vi "CRYMake Unity cal Step and unity dat.vi"(8 "Write?":bool=TRUE, 11 "Hardware flattened":string) -> (3 "Calibration flattened":string)   [LabVIEW 2013]
uses:
  Typedef Control/CRYCalibration All Cluster.ctl
  Typedef Control/CRYCalibration 2DCluster.ctl
  Typedef Control/CRYCalibration Cluster.ctl
  Typedef Control/CRYData Cluster.ctl
  CRYMainGlobal.vi
panel:
  out "output cluster":T1 {"Calibration 2D"."Sens Curve"."Z data" items=["dB", "Lin"]; "Calibration 2D"."Sens Curve"."X data" items=["dB", "Lin"]; "Calibration 2D"."Sens Curve"."Y data" items=["dB", "Lin"]; "Calibration 2D"."Sens Curve"."Z dB ref" format="%.1f"; "Calibration 2D"."Sens Curve"."Z axis" items=["Log", "Lin"]; "Calibration 2D"."Sens Curve"."X dB ref" format="%.1f"; "Calibration 2D"."Sens Curve"."X axis" items=["Log", "Lin"]; "Calibration 2D"."Sens Curve"."Y axis" items=["Log", "Lin"]; "Calibration 2D"."Sens Curve"."Y dB ref" format="%.1f"; "Calibration 2D"."Sens Curve"."Curve"."z" format="%.2f"; "Calibration 2D"."Sens Curve"."Curve"."y" format="%.2f"; "Calibration 2D"."Sens Curve"."Curve"."x" format="%.2f"; "Calibration 2D"."EQ Curve"."Z data" items=["dB", "Lin"]; "Calibration 2D"."EQ Curve"."X data" items=["dB", "Lin"]; "Calibration 2D"."EQ Curve"."Y data" items=["dB", "Lin"]; "Calibration 2D"."EQ Curve"."Z dB ref" format="%.1f"; "Calibration 2D"."EQ Curve"."Z axis" items=["Log", "Lin"]; "Calibration 2D"."EQ Curve"."X dB ref" format="%.1f"; "Calibration 2D"."EQ Curve"."X axis" items=["Log", "Lin"]; "Calibration 2D"."EQ Curve"."Y axis" items=["Log", "Lin"]; "Calibration 2D"."EQ Curve"."Y dB ref" format="%.1f"; "Calibration 2D"."EQ Curve"."Curve"."z" format="%.2f"; "Calibration 2D"."EQ Curve"."Curve"."y" format="%.2f"; "Calibration 2D"."EQ Curve"."Curve"."x" format="%.2f"; "Calibration 2D"."Corr Curve"."Z data" items=["dB", "Lin"]; "Calibration 2D"."Corr Curve"."X data" items=["dB", "Lin"]; "Calibration 2D"."Corr Curve"."Y data" items=["dB", "Lin"]; "Calibration 2D"."Corr Curve"."Z dB ref" format="%.1f"; "Calibration 2D"."Corr Curve"."Z axis" items=["Log", "Lin"]; "Calibration 2D"."Corr Curve"."X dB ref" format="%.1f"; "Calibration 2D"."Corr Curve"."X axis" items=["Log", "Lin"]; "Calibration 2D"."Corr Curve"."Y axis" items=["Log", "Lin"]; "Calibration 2D"."Corr Curve"."Y dB ref" format="%.1f"; "Calibration 2D"."Corr Curve"."Curve"."z" format="%.2f"; "Calibration 2D"."Corr Curve"."Curve"."y" format="%.2f"; "Calibration 2D"."Corr Curve"."Curve"."x" format="%.2f"; "Calibration 2D"."Calibration"."EQ Step size" items=["R10", "R20", "R40", "R80", "User"]; "Calibration 2D"."Calibration"."Corr Step size" items=["R10", "R20", "R40", "R80", "User"]}
  out "OK?":bool
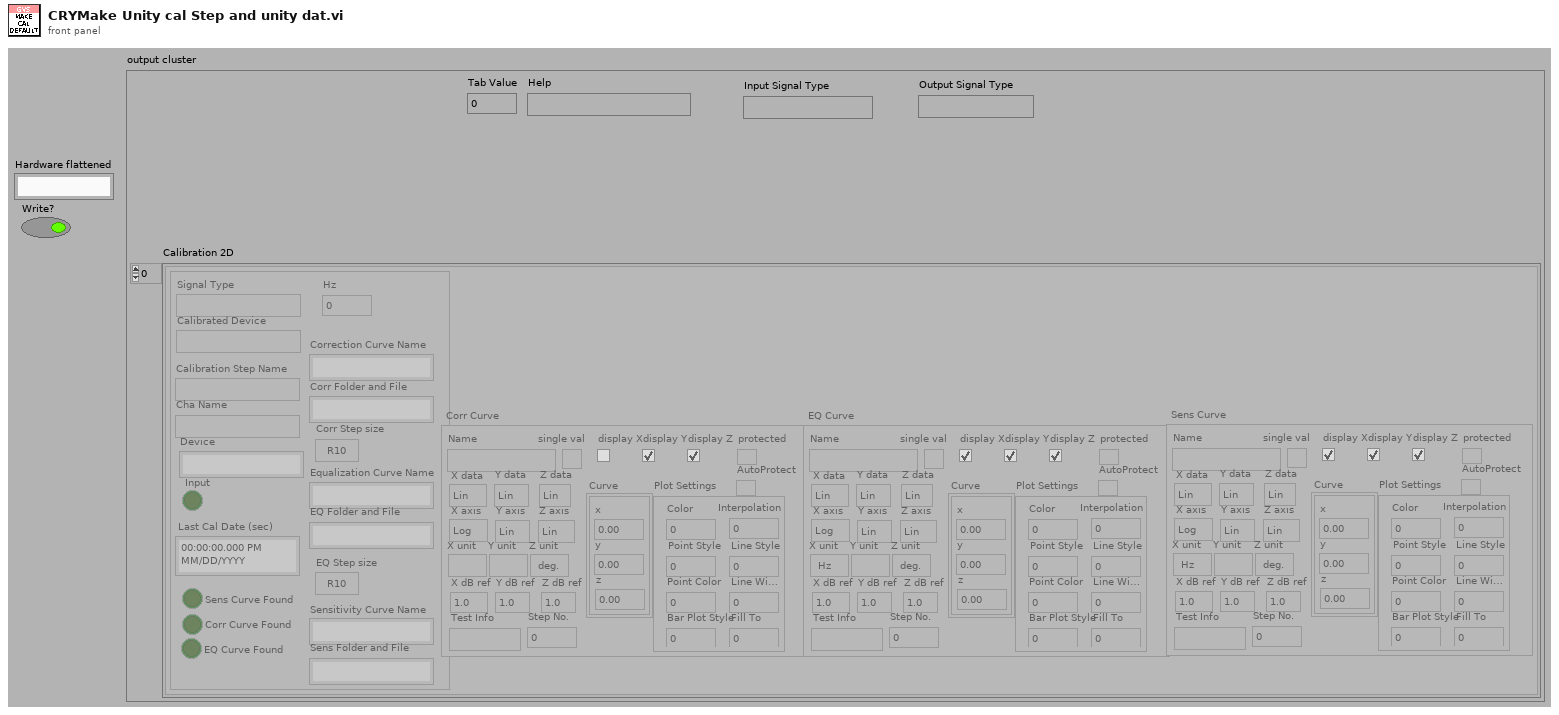
[diagram p1: front panel]
types:
  T1 = typedef "CRYCalibration All Cluster.ctl" = cluster{"Calibration 2D":T2[], "Help":string, "Tab Value":i32, "Input Signal Type":string, "Output Signal Type":string}
  T2 = typedef "CRYCalibration 2DCluster.ctl" = cluster{"Calibration":T3, "Corr Curve":T4, "EQ Curve":T4, "Sens Curve":T4}
  T3 = typedef "CRYCalibration Cluster.ctl" = cluster{"Calibration Step Name":string, "Device":string, "Correction Curve Name":string, "Equalization Curve Name":string, "Sensitivity Curve Name":string, "Corr Folder and File":string, "EQ Folder and File":string, "Sens Folder and File":string, "Corr Step size":u16, "EQ Step size":u16, "Input":bool, "Last Cal Date (sec)":timestamp, "Cha Name":string, "Corr Curve Found":bool, "EQ Curve Found":bool, "Sens Curve Found":bool, "Signal Type":string, "Calibrated Device":string, "Hz":u32}
  T4 = typedef "CRYData Cluster.ctl" = cluster{"Name":string, "Curve":cluster{"x":dbl, "y":dbl, "z":dbl}[], "X data":u16, "Y data":u16, "Z data":u16, "X axis":u16, "Y axis":u16, "Z axis":u16, "X unit":string, "Y unit":string, "Z unit":string, "X dB ref":dbl, "Y dB ref":dbl, "Z dB ref":dbl, "single val":bool, "protected":bool, "display X":bool, "display Y":bool, "display Z":bool, "Test Info":string, "Step No.":i32, "Plot Settings":cluster{"Color":u32, "Interpolation":u8, "Point Style":u8, "Line Style":u8, "Point Color":u32, "Line Width":u8, "Bar Plot Style":u8, "Fill To":i16}, "AutoProtect":bool}
  T5 = cluster{"StepName":string, "setup flattened":string}[]
  T6 = cluster{"StepName":string, "setup flattened":string}
  T7 = enum16{"open", "replace", "create", "open or create", "replace or create", "replace or create with confirmation"}
  T8 = enum16{"big-endian, network order", "native, host order", "little-endian"}
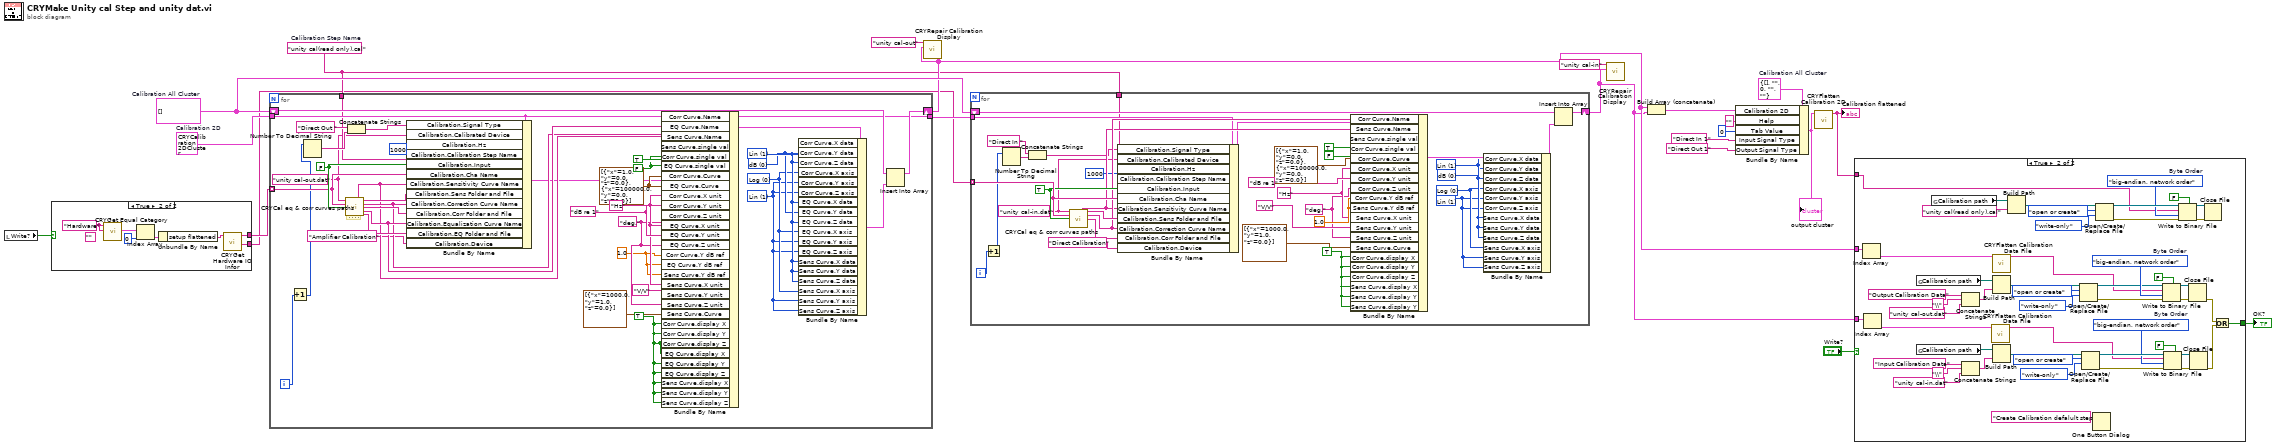
[diagram p0: block diagram]
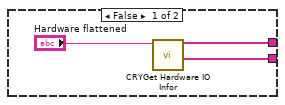
[diagram p2: hidden frame]
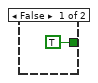
[diagram p3: hidden frame]
diagram:
  w5 = "unity cal(read only).cal"  # Calibration Step Name
  w19 = T1 {"Calibration 2D"=[], "Help"="", "Tab Value"=0, "Input Signal Type"="", "Output Signal Type"=""}  # Calibration All Cluster
  w20 = T2 {"Calibration"={"Calibration Step Name"="", "Device"="", "Correction Curve Name"="", "Equalization Curve Name"="", "Sensitivity Curve Name"="", "Corr Folder and File"="", "EQ Folder and File"="", "Sens Folder and File"="", "Corr Step size"=0, "EQ Step size"=0, "Input"=FALSE, "Last Cal Date (sec)"=timestamp(0 s since 1904-01-01), "Cha Name"="", "Corr Curve Found"=FALSE, "EQ Curve Found"=FALSE, "Sens Curve Found"=FALSE, "Signal Type"="", "Calibrated Device"="", "Hz"=0}, "Corr Curve"={"Name"="", "Curve"=[], "X data"=1, "Y data"=1, "Z data"=1, "X axis"=0, "Y axis"=1, "Z axis"=1, "X unit"="", "Y unit"="", "Z unit"="deg.", "X dB ref"=1.0, "Y dB ref"=1.0, "Z dB ref"=1.0, "single val"=FALSE, "protected"=FALSE, "display X"=FALSE, "display Y"=TRUE, "display Z"=TRUE, "Test Info"="", "Step No."=0, "Plot Settings"={"Color"=0, "Interpolation"=0, "Point Style"=0, "Line Style"=0, "Point Color"=0, "Line Width"=0, "Bar Plot Style"=0, "Fill To"=0}, "AutoProtect"=FALSE}, "EQ Curve"={"Name"="", "Curve"=[], "X data"=1, "Y data"=1, "Z data"=1, "X axis"=0, "Y axis"=1, "Z axis"=1, "X unit"="Hz", "Y unit"="", "Z unit"="deg.", "X dB ref"=1.0, "Y dB ref"=1.0, "Z dB ref"=1.0, "single val"=FALSE, "protected"=FALSE, "display X"=TRUE, "display Y"=TRUE, "display Z"=TRUE, "Test Info"="", "Step No."=0, "Plot Settings"={"Color"=0, "Interpolation"=0, "Point Style"=0, "Line Style"=0, "Point Color"=0, "Line Width"=0, "Bar Plot Style"=0, "Fill To"=0}, "AutoProtect"=FALSE}, "Sens Curve"={"Name"="", "Curve"=[], "X data"=1, "Y data"=1, "Z data"=1, "X axis"=0, "Y axis"=1, "Z axis"=1, "X unit"="Hz", "Y unit"="", "Z unit"="deg.", "X dB ref"=1.0, "Y dB ref"=1.0, "Z dB ref"=1.0, "single val"=FALSE, "protected"=FALSE, "display X"=TRUE, "display Y"=TRUE, "display Z"=TRUE, "Test Info"="", "Step No."=0, "Plot Settings"={"Color"=0, "Interpolation"=0, "Point Style"=0, "Line Style"=0, "Point Color"=0, "Line Width"=0, "Bar Plot Style"=0, "Fill To"=0}, "AutoProtect"=FALSE}}  # Calibration 2D
  w9 = T2[] []  # Calibration All Cluster
  n1 = local read "Write?"() -> (w3:bool)
  n2 = case shown="True" w3 {
    tunnel: [w23 w27] -> w2
    tunnel: [w22 w26] -> w1
    frame False {
      n3 = call "CRYGet Hardware IO Infor.vi"("Hardware setup In"="Hardware flattened") -> ("I_Hardware Channel Name Out"=w22:string[], "O_Hardware Channel Name Out"=w23:string[])  [unwired: 9 out]
    }
    frame True {
      (unwired) ""
      w25 = "Hardware" ("CategoryName")
      n4 = call "CRYGet Equal Category.vi"("Current StepName"=w25, "Find CategoryName"=w25) -> ("setup flattened Array out"=w29:T5)  [unwired: 9 out]
      n5 = Index Array(array=w29, index=0) -> (element=w30:T6)
      n6 = Unbundle By Name(w30) -> ("setup flattened"=w31:string)
      n7 = call "CRYGet Hardware IO Infor.vi"("Hardware setup In"=w31) -> ("I_Hardware Channel Name Out"=w26:string[], "O_Hardware Channel Name Out"=w27:string[])  [unwired: 9 out]
    }
  }
  n8 = for {
    tunnel: w2 -> [w37] mode=indexing
    shift-right: [w42] -> w7
    shift-left: w9 -> [w43]
    tunnel: w20 -> [w41]
    tunnel: [w41] -> w21
    tunnel: w5 -> [w33]
    i -> [w36]
    w32 = "unity cal-out.dat" ("Step Name")
    w48 = u16 1 items=["Log", "Lin"] ("Y axis")
    w49 = u16 0 items=["Log", "Lin"] ("Y axis")
    w50 = u16 0 items=["dB", "Lin"] ("Y data")
    w51 = u16 1 items=["dB", "Lin"] ("Y data")
    w52 = TRUE ("Corr Curve.display X")
    w58 = 1.0 ("EQ Curve.Y dB ref")
    w59 = "deg." ("Corr Curve.Z unit")
    w62 = "dB re 1" ("Corr Curve.Y unit")
    w61 = "Hz" ("Corr Curve.X unit")
    w63 = cluster{"x":dbl, "y":dbl, "z":dbl}[] [{"x"=1.0, "y"=0.0, "z"=0.0}, {"x"=100000.0, "y"=0.0, "z"=0.0}] ("Corr Curve.Curve")
    w64 = FALSE ("Corr Curve.single val")
    w68 = FALSE ("Input")
    # "????"
    n9 = Increment(x=w36) -> (x+1=w34:i32)
    n10 = Number To Decimal String(number=w34) -> (decimal integer string=w35:string)  [unwired: 1 in]
    n11 = call "CRYCal eq & corr curves paths.vi"("Calibrated Device Name"=w32, "Channel Name"=w37, "In_Out"=w68) -> ("Sens Currve Name"=w53:string, "Sens Curve File"=w67:string, "Corr Curve Name"=w54:string, "Corr Curve File"=w56:string, "EQ Curve Name"=w55:string, "EQ Curve File"=w66:string)  [unwired: 7 out]
    n12 = Concatenate Strings("Direct Out " ("Calibration.Signal Type"), w35) -> (w38:string)
    n13 = Bundle By Name(cluster=w41, "Calibration.Signal Type"=w38, "Calibration.Calibrated Device"=w32, "Calibration.Hz"=u32 1000, "Calibration.Calibration Step Name"=w33, "Calibration.Input"=w68, "Calibration.Cha Name"=w37, "Calibration.Sensitivity Curve Name"=w53, "Calibration.Sens Folder and File"=w67, "Calibration.Correction Curve Name"=w54, "Calibration.Corr Folder and File"=w56, "Calibration.Equalization Curve Name"=w55, "Calibration.EQ Folder and File"=w66, "Calibration.Device"="Amplifier Calibration" ("Device")) -> (w46:T2)
    n14 = Bundle By Name(cluster=w46, "Corr Curve.Name"=w54, "EQ Curve.Name"=w55, "Sens Curve.Name"=w53, "Sens Curve.single val"=TRUE, "Corr Curve.single val"=w64, "EQ Curve.single val"=w64, "Corr Curve.Curve"=w63, "EQ Curve.Curve"=w63, "Corr Curve.X unit"=w61, "Corr Curve.Y unit"=w62, "Corr Curve.Z unit"=w59, "EQ Curve.X unit"=w61, "EQ Curve.Y unit"=w62, "EQ Curve.Z unit"=w59, "Corr Curve.Y dB ref"=w58, "EQ Curve.Y dB ref"=w58, "Sens Curve.Y dB ref"=w58, "Sens Curve.X unit"=w61, "Sens Curve.Y unit"="V/V", "Sens Curve.Z unit"=w59, "Sens Curve.Curve"=cluster{"x":dbl, "y":dbl, "z":dbl}[] [{"x"=1000.0, "y"=1.0, "z"=0.0}], "Corr Curve.display X"=w52, "Corr Curve.display Y"=w52, "Corr Curve.display Z"=w52, "EQ Curve.display X"=w52, "EQ Curve.display Y"=w52, "EQ Curve.display Z"=w52, "Sens Curve.display X"=w52, "Sens Curve.display Y"=w52, "Sens Curve.display Z"=w52) -> (w45:T2)
    n15 = Bundle By Name(cluster=w45, "Corr Curve.X data"=w51, "Corr Curve.Y data"=w50, "Corr Curve.Z data"=w51, "Corr Curve.X axis"=w49, "Corr Curve.Y axis"=w48, "Corr Curve.Z axis"=w48, "EQ Curve.X data"=w51, "EQ Curve.Y data"=w50, "EQ Curve.Z data"=w51, "EQ Curve.X axis"=w49, "EQ Curve.Y axis"=w48, "EQ Curve.Z axis"=w48, "Sens Curve.X data"=w51, "Sens Curve.Y data"=w51, "Sens Curve.Z data"=w51, "Sens Curve.X axis"=w49, "Sens Curve.Y axis"=w48, "Sens Curve.Z axis"=w48) -> (w44:T2)
    n16 = Insert Into Array(array=w43, new element=w44) -> (w42:T2[])  [unwired: 1 in]
  }
  n17 = call "CRYRepair Calibration Display.vi"("Calibration In"=w7, "Calibration Step Name"="unity cal-out") -> ()  [unwired: 1 in, 9 out]
  n18 = for {
    tunnel: w1 -> [w103] mode=indexing
    tunnel: w21 -> [w81]
    shift-right: [w78] -> w6
    shift-left: w9 -> [w79]
    tunnel: w5 -> [w70]
    i -> [w76]
    w69 = "unity cal-in.dat" ("Step Name")
    w83 = u16 1 items=["Log", "Lin"] ("Y axis")
    w84 = u16 0 items=["Log", "Lin"] ("Y axis")
    w85 = u16 0 items=["dB", "Lin"] ("Y data")
    w86 = u16 1 items=["dB", "Lin"] ("Y data")
    w88 = TRUE ("Corr Curve.display X")
    w95 = 1.0 ("EQ Curve.Y dB ref")
    w92 = "deg." ("Corr Curve.Z unit")
    w94 = "Hz" ("Corr Curve.X unit")
    w102 = TRUE ("Input")
    n19 = Increment(x=w76) -> (x+1=w71:i32)
    n20 = Number To Decimal String(number=w71) -> (decimal integer string=w75:string)  [unwired: 1 in]
    n21 = Concatenate Strings("Direct In " ("string"), w75) -> (w72:string)
    n22 = call "CRYCal eq & corr curves paths.vi"("Calibrated Device Name"=w69, "Channel Name"=w103, "In_Out"=w102) -> ("Sens Currve Name"=w89:string, "Sens Curve File"=w101:string, "Corr Curve Name"=w90:string, "Corr Curve File"=w100:string)  [unwired: 9 out]
    n23 = Bundle By Name(cluster=w81, "Calibration.Signal Type"=w72, "Calibration.Calibrated Device"=w69, "Calibration.Hz"=u32 1000, "Calibration.Calibration Step Name"=w70, "Calibration.Input"=w102, "Calibration.Cha Name"=w103, "Calibration.Sensitivity Curve Name"=w89, "Calibration.Sens Folder and File"=w101, "Calibration.Correction Curve Name"=w90, "Calibration.Corr Folder and File"=w100, "Calibration.Device"="Direct Calibration" ("Device")) -> (w80:T2)
    n24 = Bundle By Name(cluster=w80, "Corr Curve.Name"=w90, "Sens Curve.Name"=w89, "Sens Curve.single val"=TRUE, "Corr Curve.single val"=FALSE, "Corr Curve.Curve"=cluster{"x":dbl, "y":dbl, "z":dbl}[] [{"x"=1.0, "y"=0.0, "z"=0.0}, {"x"=100000.0, "y"=0.0, "z"=0.0}], "Corr Curve.X unit"=w94, "Corr Curve.Y unit"="dB re 1", "Corr Curve.Z unit"=w92, "Corr Curve.Y dB ref"=w95, "Sens Curve.Y dB ref"=w95, "Sens Curve.X unit"=w94, "Sens Curve.Y unit"="V/V", "Sens Curve.Z unit"=w92, "Sens Curve.Curve"=cluster{"x":dbl, "y":dbl, "z":dbl}[] [{"x"=1000.0, "y"=1.0, "z"=0.0}], "Corr Curve.display X"=w88, "Corr Curve.display Y"=w88, "Corr Curve.display Z"=w88, "Sens Curve.display X"=w88, "Sens Curve.display Y"=w88, "Sens Curve.display Y"=w88) -> (w87:T2)
    n25 = Bundle By Name(cluster=w87, "Corr Curve.X data"=w86, "Corr Curve.Y data"=w85, "Corr Curve.Z data"=w86, "Corr Curve.X axis"=w84, "Corr Curve.Y axis"=w83, "Corr Curve.Z axis"=w83, "Sens Curve.X data"=w86, "Sens Curve.Y data"=w86, "Sens Curve.Z data"=w86, "Sens Curve.X axis"=w84, "Sens Curve.Y axis"=w83, "Sens Curve.Z axis"=w83) -> (w77:T2)
    n26 = Insert Into Array(array=w79, new element=w77) -> (w78:T2[])  [unwired: 1 in]
  }
  n27 = call "CRYRepair Calibration Display.vi"("Calibration In"=w6, "Calibration Step Name"="unity cal-in") -> ()  [unwired: 1 in, 9 out]
  n28 = Build Array (concatenate)(w7, w6) -> (w8:T2[])
  n29 = Bundle By Name(cluster=w19, "Calibration 2D"=w8, "Help"="", "Tab Value"=0, "Input Signal Type"="Direct In 1", "Output Signal Type"="Direct Out 1") -> (w18:T1)
  "output cluster" <- w18
  n30 = call "CRYFlatten Calibration 2D.vi"("Calibration All Cluster"=w18) -> ("Calibration flattened"=w4:string)  [unwired: 1 in, 9 out]
  "Calibration flattened" <- w4
  n31 = case shown="True" "Write?" {
    tunnel: w7 -> [_ w154]
    tunnel: w6 -> [_ w152]
    tunnel: [TRUE w118] -> w12
    tunnel: w4 -> [_ w107]
    frame False {
    }
    frame True {
      w109 = T8."big-endian, network order"  # Byte Order
      w124 = T8."big-endian, network order"  # Byte Order
      w149 = T8."big-endian, network order"  # Byte Order
      n32 = Index Array(array=w154) -> (element=w153:T2)  [unwired: 1 in]
      n33 = Index Array(array=w152) -> (element=w151:T2)  [unwired: 1 in]
      n34 = global read "CRYMainGlobal.vi" "Calibration path"() -> (w141:path)
      n35 = global read "CRYMainGlobal.vi" "Calibration path"() -> (w132:path)
      n36 = global read "CRYMainGlobal.vi" "Calibration path"() -> (w116:path)
      n37 = Concatenate Strings("Output Calibration Data" ("string"), "\\" ("string"), "unity cal-out.dat" ("Step File Name")) -> (w142:string)
      n38 = Concatenate Strings("Input Calibration Data" ("string"), "\\" ("string"), "unity cal-in.dat" ("Step File Name")) -> (w131:string)
      n39 = call "CRYFlatten Calibration Data File.vi"("Calibration 2D Cluster"=w151) -> ("Calibration2D flattened"=w122:string)  [unwired: 10 in]
      n40 = call "CRYFlatten Calibration Data File.vi"("Calibration 2D Cluster"=w153) -> ("Calibration2D flattened"=w121:string)  [unwired: 10 in]
      n41 = Build Path(base path=w141, name or relative path=w142) -> (appended path=w140:path)
      n42 = Build Path(base path=w132, name or relative path=w131) -> (appended path=w133:path)
      n43 = Build Path(base path=w116, name or relative path="unity cal(read only).cal" ("string")) -> (appended path=w117:path)
      n44 = Open/Create/Replace File(file path (use dialog)=w140, operation (0:open)=T7."open or create", access (0:read/write)=enum16{"read/write", "read-only", "write-only"}."write-only") -> (refnum out=w146:refnum<file>, error out=w144:errorcluster)  [unwired: 1 in, 3 out]
      n45 = Open/Create/Replace File(file path (use dialog)=w133, operation (0:open)=T7."open or create", access (0:read/write)=enum16{"read/write", "read-only", "write-only"}."write-only") -> (refnum out=w127:refnum<file>, error out=w129:errorcluster)  [unwired: 1 in, 3 out]
      n46 = One Button Dialog(message="Create Calibration defalult step") -> ()  [unwired: 2 out]
      n47 = Open/Create/Replace File(file path (use dialog)=w117, operation (0:open)=T7."open or create", access (0:read/write)=enum16{"read/write", "read-only", "write-only"}."write-only") -> (refnum out=w112:refnum<file>, error out=w114:errorcluster)  [unwired: 1 in, 3 out]
      n48 = Write to Binary File(file (use dialog)=w146, data=w121, error in=w144, 5:FALSE ("prepend array or string size? (T)"), 9:w149) -> (refnum out=w145:refnum<file>, error out=w143:errorcluster)  [unwired: 1 in, 1 out]
      n49 = Write to Binary File(file (use dialog)=w127, data=w122, error in=w129, 5:FALSE ("prepend array or string size? (T)"), 9:w124) -> (refnum out=w128:refnum<file>, error out=w130:errorcluster)  [unwired: 1 in, 1 out]
      n50 = Write to Binary File(file (use dialog)=w112, data=w107, error in=w114, 5:FALSE ("prepend array or string size? (T)"), 9:w109) -> (refnum out=w113:refnum<file>, error out=w115:errorcluster)  [unwired: 1 in, 1 out]
      n51 = Close File(refnum=w145, error in=w143) -> (error out=w120:errorcluster)  [unwired: 1 out]
      n52 = Close File(refnum=w128, error in=w130) -> (error out=w119:errorcluster)  [unwired: 1 out]
      n53 = Close File(refnum=w113, error in=w115) -> ()  [unwired: 2 out]
      n54 = Or(x=w120, y=w119) -> (x .or. y?=w118:bool)
    }
  }
  "OK?" <- w12
